vi "Get Cal Standard.vi"(11 "error in (no error)":errorcluster) -> (4 "Cal Standard Base out":refnum<class "Cal Standard Base.lvclass">, 6 "Not found":bool, 15 "error out":errorcluster)   [LabVIEW 2023, in "RFFixtureCharact.Instruments.lvlib" / "Cal Standard Factory.lvclass"]
uses:
  Cal Standard Factory/Cal Standard Factory.lvclass
  Cal Standard Base.lvclass
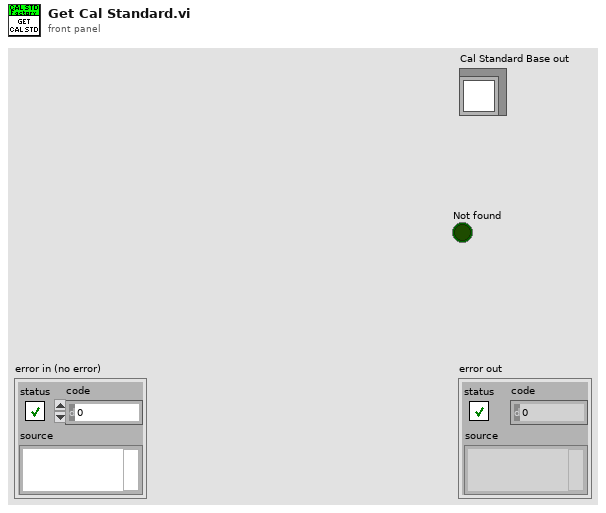
[diagram p1: front panel]
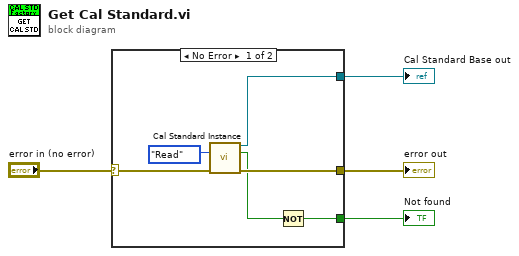
[diagram p0: block diagram]
diagram:
  n1 = case shown="No Error" "error in (no error)" {
    selector: "error in (no error)" -> [w10 w11]
    tunnel: [w9 w11] -> w2
    tunnel: [w7 _] -> w1
    tunnel: [w5 _] -> w4
    frame No Error {
      n2 = call "Cal Standard Instance.vi"("Operation"=enum16{"Read", "Write", "Clear"}."Read", "error in (no error)"=w10) -> ("Cal Standard Base out"=w7:refnum<class "Cal Standard Base.lvclass">, "Found?"=w6:bool, "error out"=w9:errorcluster)  [unwired: 11 in]
      n3 = Not(x=w6) -> (.not. x?=w5:bool)
    }
    frame Error {
    }
  }
  "error out" <- w2
  "Cal Standard Base out" <- w1
  "Not found" <- w4
